vi "RT Button Pushing.vi"() -> ()   [LabVIEW 2026]
uses:
  <vilib>/numeric/Random Number (Range) U64.vi
  <vilib>/numeric/sub_Random U32.vi
panel:
  out "Boolean":bool
  out "Numeric":i32
  in  "Stop":bool
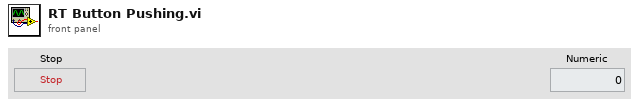
[diagram p1: front panel]
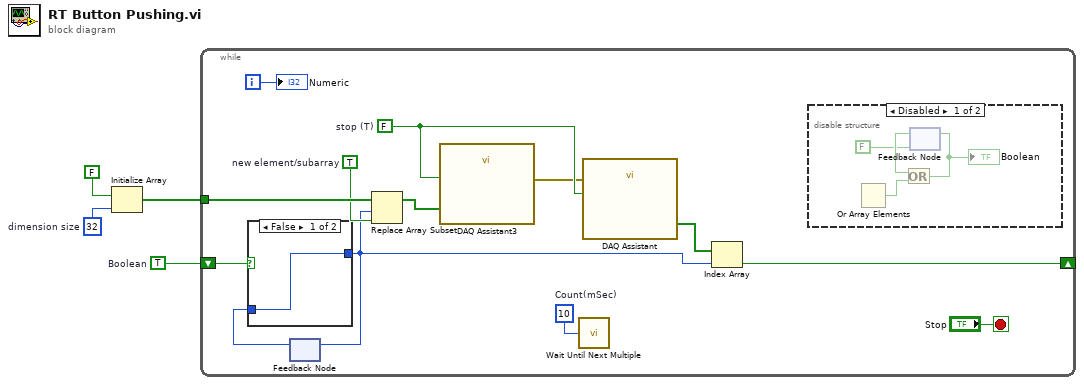
[diagram p0: block diagram]
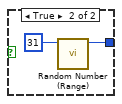
[diagram p3: hidden frame]
diagram:
  w2 = TRUE  # Boolean
  w1 = 32  # dimension size
  n1 = Initialize Array(FALSE, w1) -> (w3:bool[])
  n2 = while {
    tunnel: w3 -> [w17]
    shift-right: [w5] -> _
    shift-left: w2 -> [w14]
    i -> [w12]
    stop <- "Stop" stop-if-true
    w10 = FALSE  # stop (T)
    w7 = u32 10  # Count(mSec)
    w16 = TRUE  # new element/subarray
    n3 = feedback #1() -> (w13:u64)  [unwired: 1 in]
    n4 = case shown="False" w14 {
      tunnel: [w22 w23] -> w6
      tunnel: w13 -> [w22 _]
      frame False {
      }
      frame True {
        n5 = call-poly <vilib>:"Random Number (Range).vi"("upper bound (100)"=u64 31) -> ("number"=w23:u64)  [unwired: 10 in]
      }
    }
    n6 = feedback-in #1(w6) -> ()
    n7 = Replace Array Subset(array=w17, new element=w16, index=w6) -> (w11:bool[])
    n8 = call "DAQ Assistant3"("data"=w11, "stop (T)"=w10) -> ("error out"=w9:errorcluster)  [unwired: 16 in, 1 out]
    n9 = call "Wait Until Next Multiple"("Count(mSec)"=w7) -> ()  [unwired: 1 out]
    n10 = call "DAQ Assistant"("error in"=w9, "stop (T)"=w10) -> ("data"=w8:bool[])  [unwired: 15 in, 2 out]
    n11 = Index Array(array=w8, index=w6) -> (element=w5:bool)
    n12 = disable-structure shown="Disabled" {
      frame Disabled {
        n13 = Or Array Elements() -> (logical OR=w20:bool)  [unwired: 1 in]
        n14 = feedback #2(FALSE) -> (w21:bool)
        n15 = Or(x=w21, y=w20) -> (x .or. y?=w18:bool)
        "Boolean" <- w18
        n16 = feedback-in #2(w18) -> ()
      }
      frame Enabled {
      }
    }
    "Numeric" <- w12
  }
